vi "Receive Value Change Event.vi"(8 "error in (no error)":errorcluster, 10 "ValueChangeMsg":refnum<class "ValueChangeMsg.lvclass">, 11 "Navigation View In":refnum<class "Navigation View.lvclass">) -> (0 "error out":errorcluster, 3 "Navigation View Out":refnum<class "Navigation View.lvclass">)   [LabVIEW 2019, in "Navigation View.lvclass"]
doc: "<License>\nCopyright © 2017 Composed Systems, LLC | All rights reserved\nwww.composed.io\n\nAuthor: Ethan Stern <ethan.stern@composed.io>\n\nThis software is provided \"AS IS\" WITHOUT WARRANTIES, either express or implied, AND IS FOR EDUCATIONAL PURPOSES ONLY.\n</License>"
uses:
  <vilib>/gpm_packages/@cs/Car-wash/Source/Navigation View/Navigation View.lvclass
  <vilib>/gpm_packages/@cs/mva-viewable/Source/ActorEvents/IEventAggregator Messages/ValueChangeMsg/ValueChangeMsg.lvclass
  <vilib>/gpm_packages/@cs/mva-viewable/Source/ActorEvents/IEventAggregator Messages/ValueChangeMsg/ValueChangeMsg.lvclass/ValueChangeMsg.ctl
  <vilib>/gpm_packages/@cs/Car-wash/Source/Navigation View/Navigation View.lvclass/Navigation View.ctl
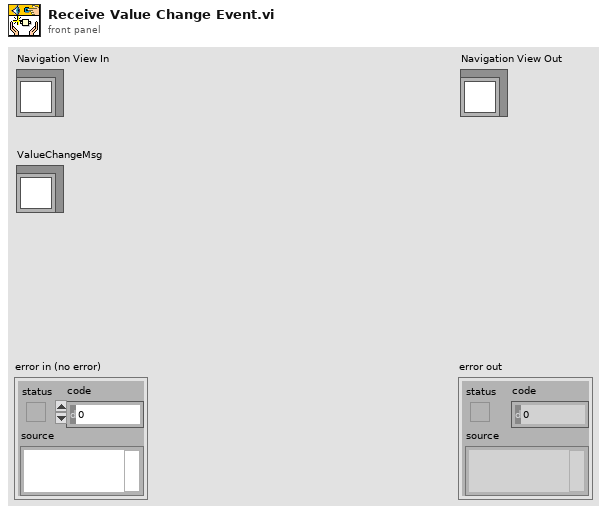
[diagram p1: front panel]
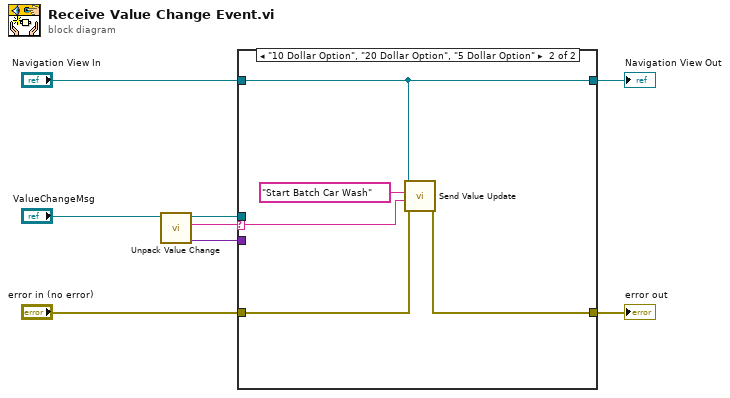
[diagram p0: block diagram]
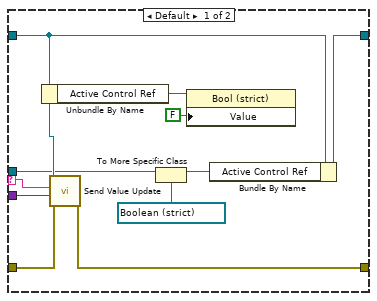
[diagram p2: hidden frame]
diagram:
  n1 = call <vilib>:"Unpack Value Change.vi"("ValueChangeMsg"="ValueChangeMsg") -> ("New Value"=w4:variant, "Control Label"=w5:string, "Ctl Refnum"=w1:refnum<vi>)  [unwired: 6 in, 2 out]
  n2 = case shown="\"10 Dollar Option\", \"20 Dollar Option\", \"5 Dollar Option\"" w5 {
    selector: w5 -> [w19 w22]
    tunnel: "error in (no error)" -> [w17 w21]
    tunnel: "Navigation View In" -> [w13 w24]
    tunnel: w4 -> [w18 _]
    tunnel: [w12 w24] -> w3
    tunnel: [w16 w20] -> w2
    tunnel: w1 -> [w11 _]
    frame Default {
      n3 = Unbundle By Name(w13) -> ("Active Control Ref"=w15:refnum<vi>)
      n4 = call-dynamic "Send Value Update.vi"("error in (no error)"=w17, "Value"=w18, "Datum Name"=w19, "IViewable in"=w13) -> ("error out"=w16:errorcluster)  [unwired: 7 in]
      n5 = To More Specific Class(target class=refnum<vi> refnum ("Active Control Ref"), reference=w11) -> (specific class reference=w10:refnum<vi>)  [unwired: 1 in, 1 out]
      n6 = property class="Bool (strict)"(reference=w15, "Value"=FALSE) -> ()  [unwired: 1 in, 2 out]
      n7 = Bundle By Name(cluster=w13, "Active Control Ref"=w10) -> (w12:refnum<class "Navigation View.lvclass">)
    }
    frame "10 Dollar Option", "20 Dollar Option", "5 Dollar Option" {
      n8 = call-dynamic "Send Value Update.vi"("error in (no error)"=w21, "Value"=w22, "Datum Name"="Start Batch Car Wash", "IViewable in"=w24) -> ("error out"=w20:errorcluster)  [unwired: 7 in]
    }
  }
  "error out" <- w2
  "Navigation View Out" <- w3
